vi "Type Color.vi"(11 "ColumnPanel in":refnum<class "ColumnPanel.lvclass">) -> (2 "Type Color":u32(colorbox))   [LabVIEW 2020, in "Conditum-Tools.lvlib" / "ColumnPanel.lvclass"]
uses:
  ColumnPanel.lvclass
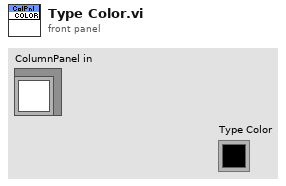
[diagram p1: front panel]
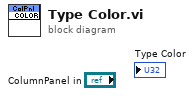
[diagram p0: block diagram]
diagram:
